vi "ASCII to HEX.vi"(10 "ASCII String":string="5051525354A5A6A7A8A9") -> (2 "Hex String":string)   [LabVIEW 2016]
panel:
  out "byte count":u32=1200
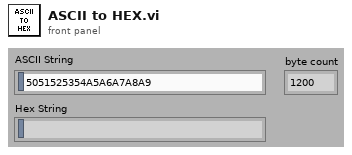
[diagram p1: front panel]
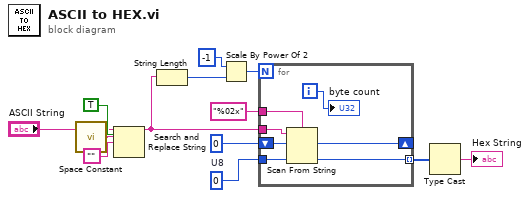
[diagram p0: block diagram]
diagram:
  w12 = u8 0  # U8
  n1 = call <vilib>:"Space Constant.vi"() -> ("String"=w3:string)
  n2 = Search and Replace String(replace all?=TRUE, input string="ASCII String", search string=w3, replace string="") -> (result string=w1:string)  [unwired: 4 in, 3 out]
  n3 = String Length(string=w1) -> (length=w9:i32)
  n4 = Scale By Power Of 2(n=-1, x=w9) -> (x*2^n=w7:i32)
  n5 = for {
    N: w7 -> [_]
    shift-right: [w19] -> _
    shift-left: u32 0 -> [w20]
    tunnel: w1 -> [w16]
    tunnel: w12 -> [w18]
    tunnel: [w15] -> w11 mode=indexing
    tunnel: "%02x" ("format string") -> [w17]
    i -> [w14]
    n6 = Scan From String(format string=w17, input string=w16, initial scan location=w20, default 1=w18) -> (offset past scan=w19:u32, output 1=w15:u8)  [unwired: 1 in, 2 out]
    "byte count" <- w14
  }
  n7 = Type Cast(x=w11) -> (*(type *) &x=→"Hex String":string)  [unwired: 1 in]
